vi "Test.Maui 2.0.Initialize.Scarce.Rings.Ring 1.vi"(8 "error in":errorcluster) -> (0 "error out":errorcluster)   [LabVIEW 2020]
uses:
  Maui 2.0/Maui 2.0.lvclass
  C:/Program Files (x86)/National Instruments/LabVIEW 2020/vi.lib/JKI/JKI SMO/SMO/SMO.lvclass
  Helper/Test Helper 1/Test Helper 1.lvclass
  <vilib>/addons/_JKI Toolkits/Caraya/classes/Assert/Assert Equal Value_Variant.vi
  <vilib>/addons/_JKI Toolkits/Caraya/classes/Assert/Assert True.vi
  <vilib>/JKI/JKI SMO/SMO/SMO.lvclass
  <vilib>/addons/_JKI Toolkits/Caraya/classes/Assert/Assert.lvclass
  <vilib>/addons/_JKI Toolkits/Caraya/classes/Test/Test.lvclass
panel:
  in  "Ring 2":u16(ring) items=["Test Helper 1", "None"]
  in  "Ring":u16(ring) items=["Test Helper 1", "None"]
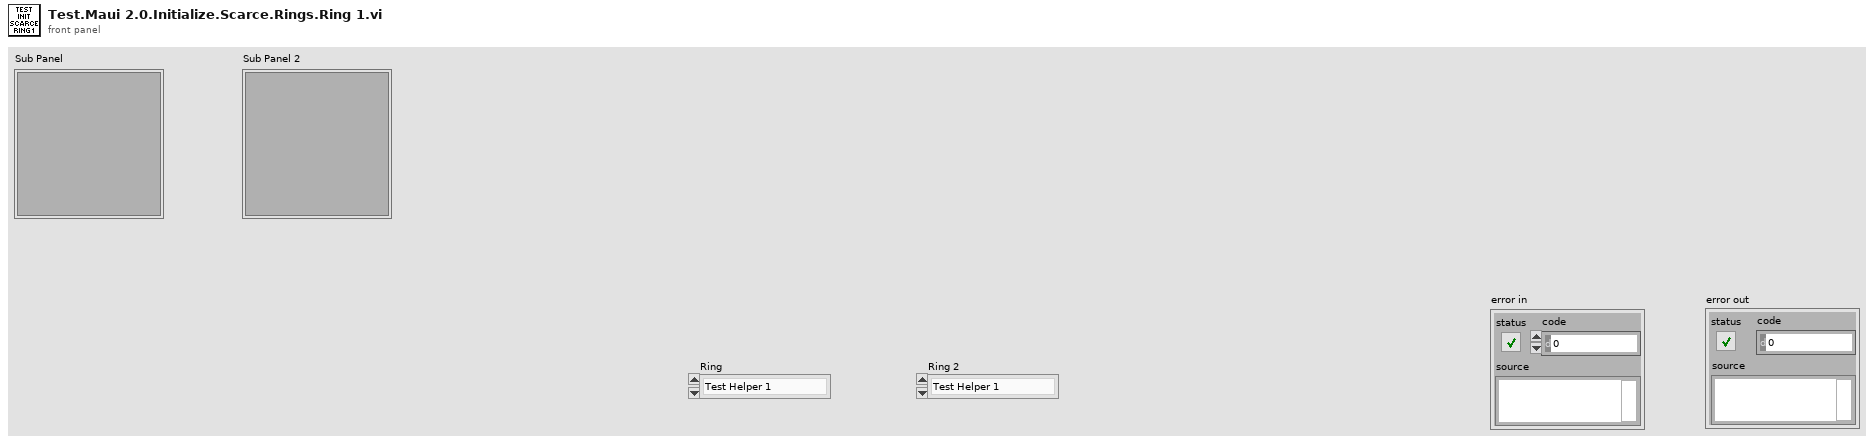
[diagram p1: front panel]
types:
  T1 = cluster{"Ring":refnum<vi>, "Sub Panel":refnum<vi>}
  T2 = cluster{"Ring 2":refnum<vi>, "Sub Panel 2":refnum<vi>}
  T3 = cluster{"Ring 2":refnum<vi>, "Sub Panel 2":refnum<vi>}[]
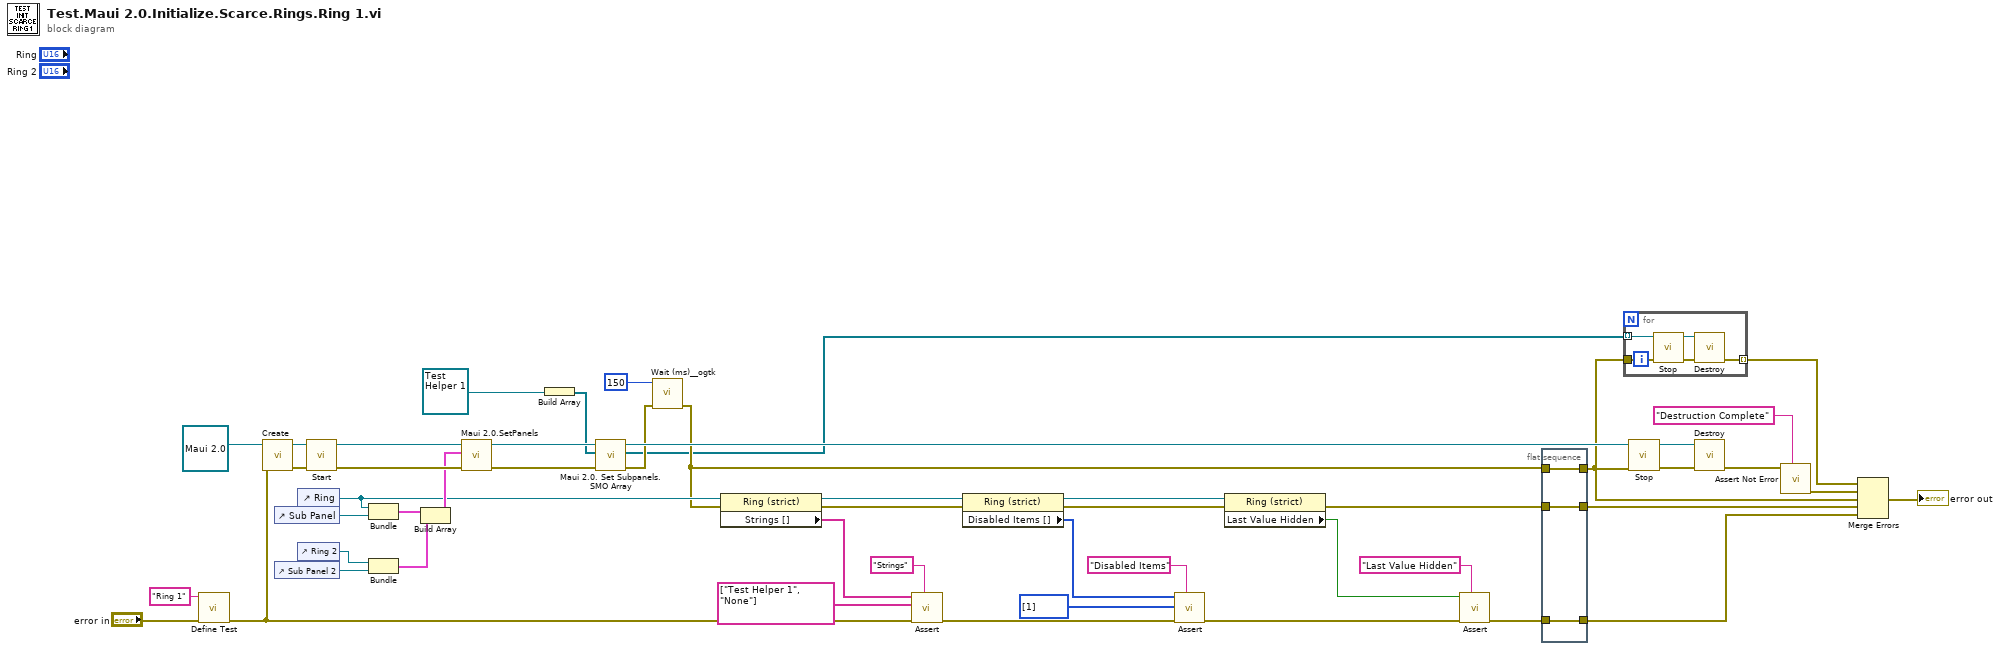
[diagram p0: block diagram]
diagram:
  n1 = call <vilib>:"Define Test.vi"("error in (no error)"="error in", "Label (VI Title)"="Ring 1") -> ("error out"=w25:errorcluster)  [unwired: 9 in]
  n2 = call <vilib>:"Create.vi"("error in (no error)"=w25, "SMO"=refnum<class "Maui 2.0.lvclass"> refnum ("Maui 2.0 in")) -> ("error out"=w50:errorcluster, "SMO out"=w42:refnum<class "Maui 2.0.lvclass">)  [unwired: 7 in, 1 out]
  n3 = control-ref of="Sub Panel"() -> (w47:refnum<vi>)
  n4 = control-ref of="Sub Panel 2"() -> (w45:refnum<vi>)
  n5 = control-ref of="Ring"() -> (w35:refnum<vi>)
  n6 = control-ref of="Ring 2"() -> (w46:refnum<vi>)
  n7 = call <vilib>:"Start.vi"("error in (no error)"=w50, "SMO"=w42) -> ("error out"=w49:errorcluster, "SMO out"=w40:refnum<class "Maui 2.0.lvclass">)  [unwired: 8 in]
  n8 = Bundle("Ring"=w35, "Sub Panel"=w47) -> (w44:T1)  [unwired: 1 in]
  n9 = Bundle("Ring 2"=w46, "Sub Panel 2"=w45) -> (w43:T2)  [unwired: 1 in]
  n10 = Build Array(w44, w43) -> (w36:T3)
  n11 = call "Maui 2.0.SetPanels.vi"("error in (no error)"=w49, "Set Panels"=w36, "Maui 2.0"=w40) -> ("error out"=w48:errorcluster, "Maui 2.0 out"=w39:refnum<class "Maui 2.0.lvclass">)  [unwired: 7 in]
  n12 = Build Array(refnum<class "Test Helper 1.lvclass"> refnum ("Test Helper 1.lvclass")) -> (w37:refnum<class "Test Helper 1.lvclass">[])
  n13 = call-dynamic "Maui 2.0. Set Subpanels.SMO Array.vi"("error in (no error)"=w48, "Subpanels in"=w37, "Maui 2.0 in"=w39) -> ("error out"=w9:errorcluster, "Subpanels Out"=w6:refnum<class "SMO.lvclass">[], "Maui 2.0 out"=w19:refnum<class "Maui 2.0.lvclass">)  [unwired: 6 in]
  n14 = call <userlib>:"Wait (ms)__ogtk.vi"("error in (no error)"=w9, "milliseconds to wait"=u32 150) -> ("error out"=w8:errorcluster)  [unwired: 8 in, 1 out]
  n15 = property class="Ring (strict)"(reference=w35, error in=w8) -> (reference out=w29:refnum<vi>, error out=w22:errorcluster, "Strings []"=w33:string[])
  n16 = call-poly <vilib>:"Assert.vi"("Label"="Strings", "error in (no error)"=w25, "Y"=string[] ["Test Helper 1", "None"], "X"=w33) -> ("error out"=w23:errorcluster)  [unwired: 7 in]
  n17 = property class="Ring (strict)"(reference=w29, error in=w22) -> (reference out=w27:refnum<vi>, error out=w21:errorcluster, "Disabled Items []"=w3:i32[])
  n18 = call-poly <vilib>:"Assert.vi"("Label"="Disabled Items", "error in (no error)"=w23, "Y"=i32[] [1] ("Disabled Items []"), "X"=w3) -> ("error out"=w24:errorcluster)  [unwired: 7 in]
  n19 = property class="Ring (strict)"(reference=w27, error in=w21) -> (error out=w13:errorcluster, "Last Value Hidden"=w20:bool)  [unwired: 1 out]
  n20 = call-poly <vilib>:"Assert.vi"("Label"="Last Value Hidden", "error in (no error)"=w24, "True?"=w20) -> ("error out"=w12:errorcluster)  [unwired: 8 in]
  n21 = flat-sequence {
    tunnel: w8 -> [w53]
    tunnel: w13 -> [w52]
    tunnel: w12 -> [w51]
    tunnel: [w53] -> w4
    tunnel: [w52] -> w11
    tunnel: [w51] -> w10
    frame #0 {
    }
  }
  n22 = for {
    tunnel: w6 -> [w57] mode=indexing
    tunnel: w4 -> [w56]
    tunnel: [w54] -> w5 mode=indexing
    n23 = call <vilib>:"Stop.vi"("error in (no error)"=w56, "SMO"=w57) -> ("error out"=w55:errorcluster, "SMO out"=w58:refnum<class "SMO.lvclass">)  [unwired: 8 in]
    n24 = call <vilib>:"Destroy.vi"("error in (no error)"=w55, "SMO"=w58) -> ("error out"=w54:errorcluster)  [unwired: 9 in]
  }
  n25 = call <vilib>:"Stop.vi"("error in (no error)"=w4, "SMO"=w19) -> ("error out"=w17:errorcluster, "SMO out"=w18:refnum<class "Maui 2.0.lvclass">)  [unwired: 8 in]
  n26 = call <vilib>:"Destroy.vi"("error in (no error)"=w17, "SMO"=w18) -> ("error out"=w16:errorcluster)  [unwired: 9 in]
  n27 = call <vilib>:"Assert Not Error.vi"("Label"="Destruction Complete", "Not Error?"=w16) -> ("error out"=w14:errorcluster)  [unwired: 9 in]
  n28 = Merge Errors(w5, w14, w4, w11, w10) -> (→"error out":errorcluster)
